vi "GFITS_inspectErros.vi"(7 "message":string, 8 "error in (no error)":errorcluster, 10 "errno str":string, 11 "error code":i32) -> (0 "error out":errorcluster)   [LabVIEW 2016]
doc: "This subVI tests the error status output of one or more low-level functions or subVIs that output a numeric error code, and creates an error out cluster that can be wired to the Simple or General Error Handler in order to identify the error and describe it to the user.\n\nThe error in cluster is tested first. If error? is no-error, the elements of the error codes array are tested next for non-zero values. The first error found terminates the test, and error out identifies that error. Use a Build Array function to assemble the individual error codes.\n\nYou can optionally use the source messages string to pass on the source of the error. Enter one line of text for each element of the error codes array. \n\nThe error? status is TRUE on any error."
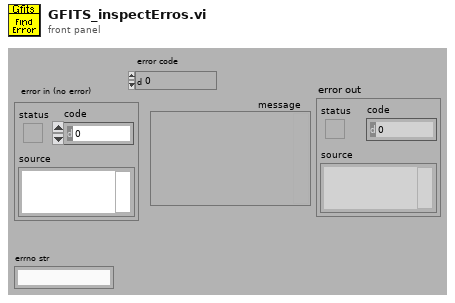
[diagram p1: front panel]
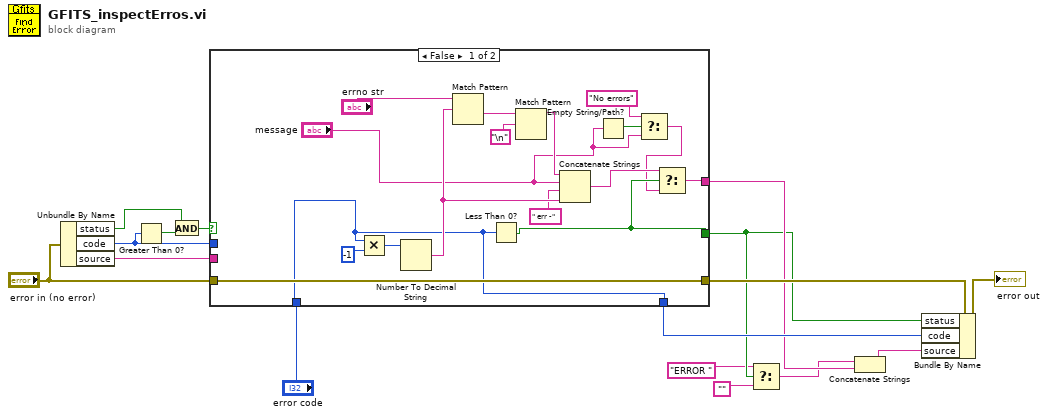
[diagram p0: block diagram]
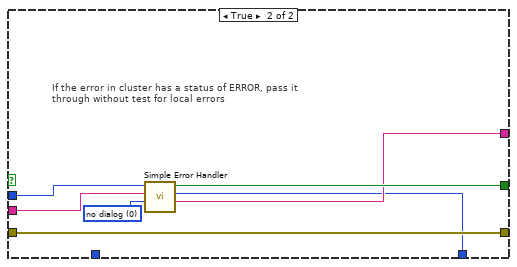
[diagram p2: hidden frame]
diagram:
  n1 = Unbundle By Name("error in (no error)") -> ("status"=w3:bool, "code"=w2:i32, "source"=w15:string)
  n2 = Greater Than 0?(x=w2) -> (x > 0?=w1:bool)
  n3 = And(x=w3, y=w1) -> (x .and. y?=w4:bool)
  n4 = case shown="False" w4 {
    tunnel: "error in (no error)" -> [w33 w40]
    tunnel: [w33 w40] -> w14
    tunnel: [w23 w37] -> w10
    tunnel: [w21 w38] -> w8
    tunnel: w2 -> [_ w36]
    tunnel: w15 -> [_ w39]
    tunnel: "error code" -> [w22 _]
    tunnel: [w22 w35] -> w11
    frame False {
      n5 = Multiply(x=w22, y=-1) -> (x*y=w26:i32)
      n6 = Number To Decimal String(number=w26) -> (decimal integer string=w29:string)  [unwired: 1 out]
      n7 = Match Pattern(string="errno str", regular expression=w29) -> (after substring=w31:string)  [unwired: 4 out]
      n8 = Less Than 0?(x=w22) -> (x < 0?=w21:bool)
      n9 = Match Pattern(string=w31, regular expression="\n") -> (before substring=w27:string)  [unwired: 4 out]
      n10 = Concatenate Strings(w27, "message", " err -", w29) -> (w24:string)
      n11 = Empty String/Path?(string/path="message") -> (empty?=w20:bool)
      n12 = Select(t="No errors", s=w20, f="message") -> (s? t:f=w18:string)
      n13 = Select(t=w24, s=w21, f=w18) -> (s? t:f=w23:string)
    }
    frame True {
      w34 = u16 0 items=["no dialog", "OK message", "continue or stop message"] ("type of dialog (OK msg:1)")
      # "If the error in cluster has a status of ERROR, pass it through without test for local errors"
      n14 = call <vilib>:"Simple Error Handler.vi"("error code (no error:0)"=w36, "error source (\" \")"=w39, "type of dialog (OK msg:1)"=w34) -> ("error?"=w38:bool, "code out"=w35:i32, "source out"=w37:string)  [unwired: 1 in, 3 out]
    }
  }
  n15 = Select(t="ERROR ", s=w8, f="") -> (s? t:f=w5:string)
  n16 = Concatenate Strings(w5, w10) -> (w9:string)
  n17 = Bundle By Name(cluster=w14, "status"=w8, "code"=w11, "source"=w9) -> (→"error out":errorcluster)
